vi "Laser 1 Operations L2.vi"(8 "Error in":errorcluster caption="Error in (no error)", 10 "Queues Cluster":T1, 11 "UI elements cluster":T2) -> (0 "Error out":errorcluster)   [LabVIEW 2017]
uses:
  Global Variables/General Globals.vi
  Typedefs/XY Stage config cluster.ctl
  Typedefs/Cam VidRec HW config setup cluster.ctl
  Typedefs/Control Sys HW config cluster.ctl
  <vilib>/userdefined/High Color/nirio_resource_hc.ctl
  Typedefs/FPGA input type AC-DC.ctl
  Typedefs/DAQmx physical channels cluster.ctl
  Typedefs/Encoder config cluster.ctl
  Typedefs/Z Stage config cluster.ctl
  Typedefs/Triggers HW config.ctl
  Typedefs/Laser 1 config cluster.ctl
  Typedefs/PreChirper 1 config cluster.ctl
  Typedefs/Microscope Config.ctl
  Typedefs/Laser Power Control HW config.ctl
  Typedefs/Hardware Configuration settings.ctl
  Serial Comms/Visa resource.ctl
  Typedefs/Plane Mode.ctl
  Typedefs/Laser control knob.ctl
  Typedefs/PMT control knob.ctl
  Typedefs/XY Stage_Move.ctl
  Typedefs/Frame Size.ctl
  Typedefs/UI ctrl refs cluster.ctl
  Typedefs/Imaging Param ref.ctl
  User Interface/Queue/Message Queue/Typedefs/Message Cluster.ctl
  Typedefs/Imaging Protocols enum.ctl
  Typedefs/Acquired points count.ctl
  Typedefs/Logging queue element.ctl
  User Interface/Queue/Message Queue/Typedefs/All Message Queues.ctl
panel:
  in  "Wavelength \n(set) [nm]":u16
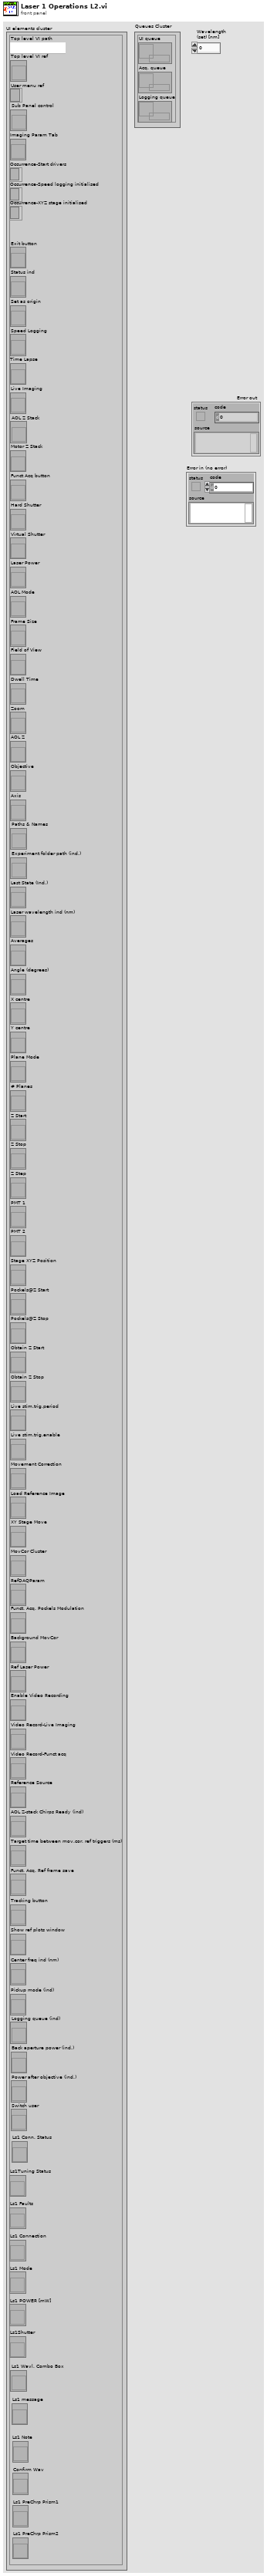
[diagram p1: front panel]
types:
  T1 = typedef "All Message Queues.ctl" = cluster{"UI queue":refnum<queue>, "Acq. queue":refnum<queue>, "Logging queue":refnum<queue>}
  T2 = typedef "UI ctrl refs cluster.ctl" = cluster{"Top level VI path":path, "Top level VI ref":refnum<vi>, "User menu ref":refnum<k9>, "Sub Panel control":refnum<vi>, "Imaging Param Tab":T3, "Occurrence-Start drivers":refnum<k4>, "Occurrence-Speed logging initialised":refnum<k4>, "Occurrence-XYZ stage initialised":refnum<k4>, "Exit button":refnum<vi>, "Status ind":refnum<vi>, "Set as origin":refnum<vi>, "Speed Logging":refnum<vi>, "Time Lapse":refnum<vi>, "Live Imaging":refnum<vi>, "AOL Z Stack":refnum<vi>, "Motor Z Stack":refnum<vi>, "Funct Acq button":refnum<vi>, "Hard Shutter":refnum<vi>, "Virtual Shutter":refnum<vi>, "Laser Power":refnum<vi>, "AOL Mode":refnum<vi>, "Frame Size":refnum<vi>, "Field of View":refnum<vi>, "Dwell Time":refnum<vi>, "Zoom":refnum<vi>, "AOL Z":refnum<vi>, "Objective":refnum<vi>, "Axis":refnum<vi>, "Paths & Names":refnum<vi>, "Experiment folder path (ind.)":refnum<vi>, "Last State (Ind.)":refnum<vi>, "Laser wavelength ind (nm)":refnum<vi>, "Averages":refnum<vi>, "Angle (degrees)":refnum<vi>, "X centre":refnum<vi>, "Y centre":refnum<vi>, "Plane Mode":refnum<vi>, "# Planes":refnum<vi>, "Z Start":refnum<vi>, "Z Stop":refnum<vi>, "Z Step":refnum<vi>, "PMT 1":refnum<vi>, "PMT 2":refnum<vi>, "Stage XYZ Position":refnum<vi>, "Pockels@Z Start":refnum<vi>, "Pockels@Z Stop":refnum<vi>, "Obtain Z Start":refnum<vi>, "Obtain Z Stop":refnum<vi>, "Live stim.trig.period":refnum<vi>, "Live stim.trig.enable":refnum<vi>, "Movement Correction":refnum<vi>, "Load Reference Image":refnum<vi>, "XY Stage Move":refnum<vi>, "MovCor Cluster":refnum<vi>, "RefDAQParam":refnum<vi>, "Funct. Acq. Pockels Modulation":refnum<vi>, "Background MovCor":refnum<vi>, "Ref Laser Power":refnum<vi>, "Enable Video Recording":refnum<vi>, "Video Record-Live Imaging":refnum<vi>, "Video Record-Funct acq":refnum<vi>, "Reference Source":refnum<vi>, "AOL Z-stack Chirps Ready (ind)":refnum<vi>, "Target time between mov.cor. ref triggers (ms)":refnum<vi>, "Funct. Acq. Ref frame save":refnum<vi>, "Tracking button":refnum<vi>, "Show ref plots window":refnum<vi>, "Center freq ind (nm)":refnum<vi>, "Pickup mode (ind)":refnum<vi>, "Logging queue (ind)":refnum<vi>, "Back aperture power (ind.)":refnum<vi>, "Power after objective (ind.)":refnum<vi>, "Switch user":refnum<vi>, "Ls1 Conn. Status":refnum<vi>, "Ls1Tuning Status":refnum<vi>, "Ls1 Faults":refnum<vi>, "Ls1 Connection":refnum<vi>, "Ls1 Mode":refnum<vi>, "Ls1 POWER [mW]":refnum<vi>, "Ls1Shutter":refnum<vi>, "Ls1 Wavl. Combo Box":refnum<vi>, "Ls1 message":refnum<vi>, "Ls1 Note":refnum<vi>, "Confirm Wav":refnum<vi>, "Ls1 PreChrp Prism1":refnum<vi>, "Ls1 PreChrp Prism2":refnum<vi>}
  T3 = typedef "Imaging Param ref.ctl" = refnum<vi>
  T4 = typedef "Hardware Configuration settings.ctl" = cluster{"Computer MAC address":string, "XY Stage":T5, "Cam VidRec":T6, "Control Sys. HW config":T7, "DAQ FPGA HW Config":cluster{"Target":T8, "input card type":T9}, "DAQmx Chan":T10, "Encoder":T11, "Z Stage config cluster":T12, "Trigger HW config":T13, "Externalise Triggers":bool, "MC Supported":bool, "Laser 1 config cluster":T14, "Prechirper 1 config cluster":T15, "Microscope Config":T16, "Laser Power Control HW config":T17, "No of AOD":u8, "Dev. PC":bool}
  T5 = typedef "XY Stage config cluster.ctl" = cluster{"COM port":refnum<visa-resource-name>, "XY stage available":bool, "Baudrate":i32, "Type":string}
  T6 = typedef "Cam VidRec HW config setup cluster.ctl" = cluster{"DO flag-Video record":tag, "DO flag-Trial start":tag, "VidRec available":bool}
  T7 = typedef "Control Sys HW config cluster.ctl" = cluster{"Ctrl system MAC address":string, "Control system.Network adapter name":string, "Ctrl FPGA available":bool}
  T8 = typedef "nirio_resource_hc.ctl" = tag
  T9 = typedef "FPGA input type AC-DC.ctl" = enum16{"AC Card", "DC Card"}
  T10 = typedef "DAQmx physical channels cluster.ctl" = cluster{"Pockels AO":tag, "Hard shutter AO":tag, "PMT AOs":tag, "Power meter AI":tag}
  T11 = typedef "Encoder config cluster.ctl" = cluster{"IP address":string, "Port":u16, "Encoder available":bool, "Wheel radius (cm)":dbl}
  T12 = typedef "Z Stage config cluster.ctl" = cluster{"COM port":refnum<visa-resource-name>, "Z stage available":bool, "Baudrate":i32, "Type":string}
  T13 = typedef "Triggers HW config.ctl" = cluster{"Available Device List":i32, "Device Address":string}
  T14 = typedef "Laser 1 config cluster.ctl" = cluster{"COM port":refnum<visa-resource-name>, "Laser 1 available":bool, "Baud Rate":i32, "Type":string}
  T15 = typedef "PreChirper 1 config cluster.ctl" = cluster{"COM port":refnum<visa-resource-name>, "Prechirper 1 \navailable":bool, "Baud Rate":i32, "Type":string}
  T16 = typedef "Microscope Config.ctl" = cluster{"ID":string, "Type":string}
  T17 = typedef "Laser Power Control HW config.ctl" = cluster{"Laser Power Control":string, "Laser Power Modulation Control":string}
  T18 = enum16{"Initialise Connections", "Initialise system", "Check Status", "Open/Close Shutter", "Set wavelength", "Close"}
  T19 = typedef "Visa resource.ctl" = cluster{"VISA resource name":refnum<visa-resource-name>, "baud rate":u32}
  T20 = enum16{"Initialise", "Disable Controls", "Enable Controls", "Update Connection Info", "Update Laser Warning", "Update Laser status", "Update Laser Wav.", "Update prechiper settings"}
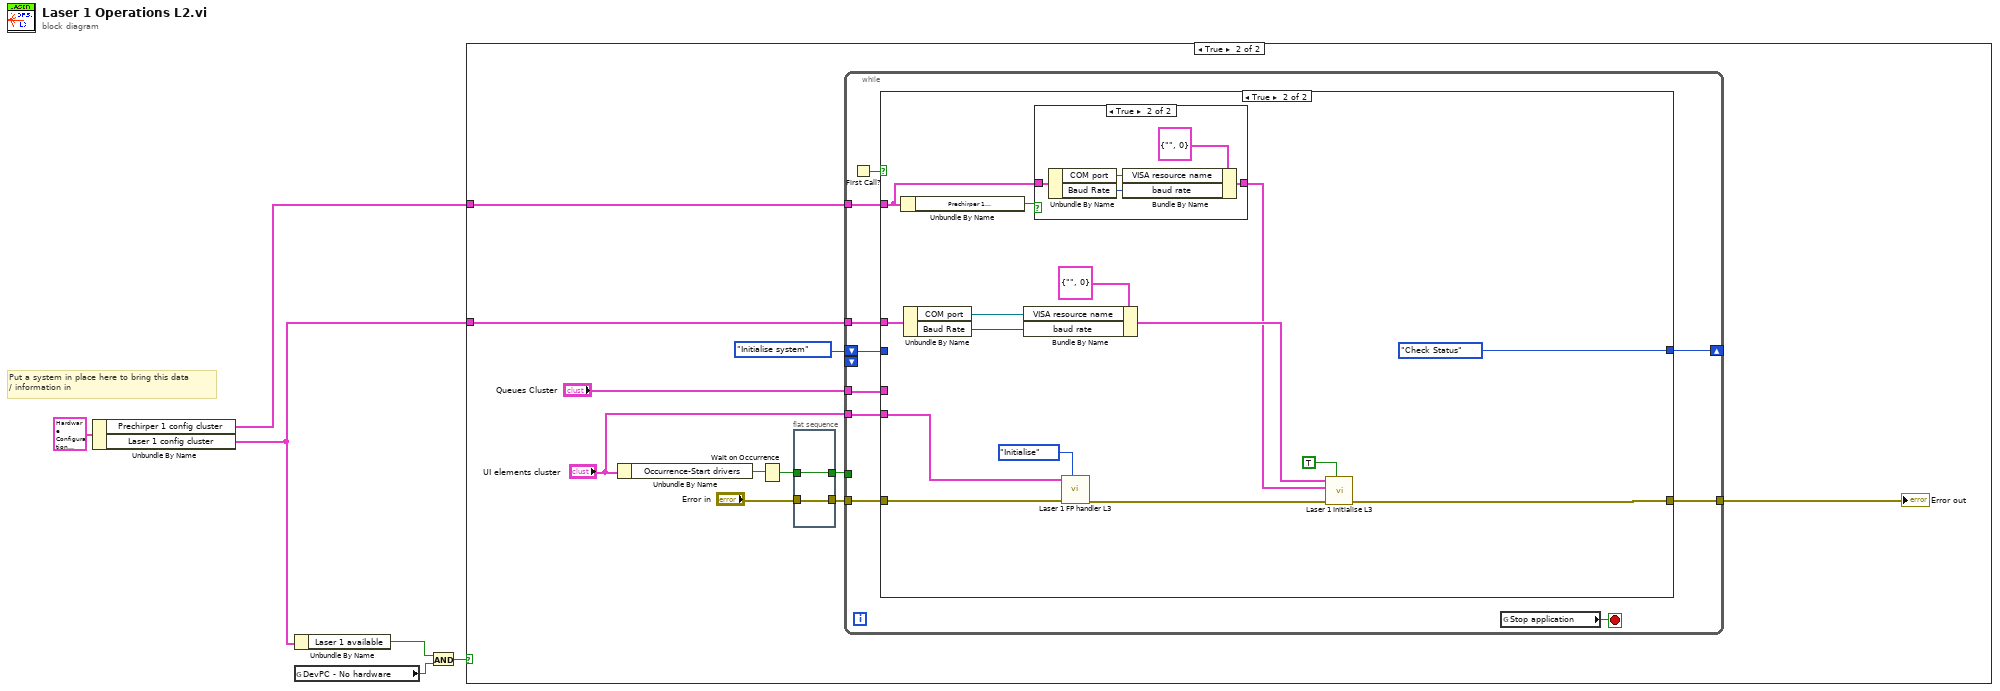
[diagram p0: block diagram]
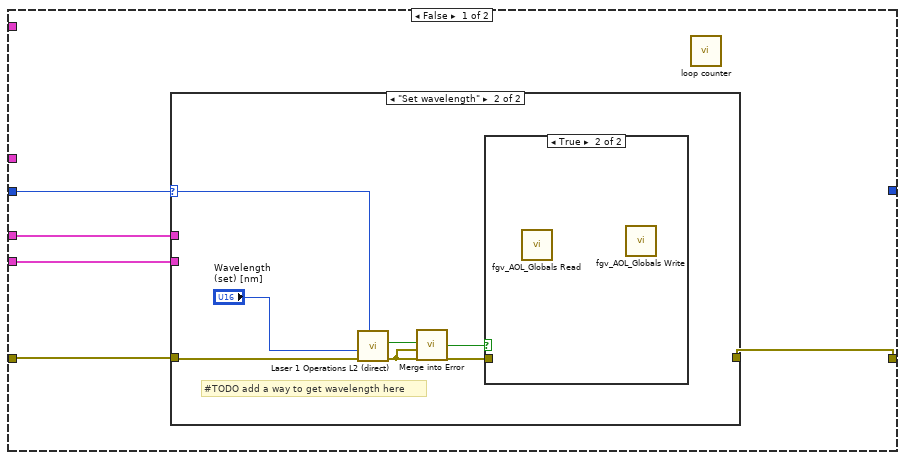
[diagram p3: hidden frame]
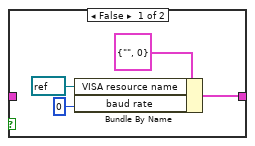
[diagram p6: hidden frame]
diagram:
  # "Put a system in place here to bring this data\n/ information in"
  n1 = Unbundle By Name(T4 {"Computer MAC address"="", "XY Stage"={"COM port"="", "XY stage available"=FALSE, "Baudrate"=0, "Type"=""}, "Cam VidRec"={"DO flag-Video record"="", "DO flag-Trial start"="", "VidRec available"=FALSE}, "Control Sys. HW config"={"Ctrl system MAC address"="", "Control system.Network adapter name"="", "Ctrl FPGA available"=FALSE}, "DAQ FPGA HW Config"={"Target"="RIO0", "input card type"=enum."AC Card"}, "DAQmx Chan"={"Pockels AO"="", "Hard shutter AO"="", "PMT AOs"="", "Power meter AI"=""}, "Encoder"={"IP address"="224.0.1.103", "Port"=7000, "Encoder available"=FALSE, "Wheel radius (cm)"=16.0}, "Z Stage config cluster"={"COM port"="COM7", "Z stage available"=FALSE, "Baudrate"=0, "Type"=""}, "Trigger HW config"={"Available Device List"=0, "Device Address"=""}, "Externalise Triggers"=FALSE, "MC Supported"=FALSE, "Laser 1 config cluster"={"COM port"="COM7", "Laser 1 available"=FALSE, "Baud Rate"=0, "Type"=""}, "Prechirper 1 config cluster"={"COM port"="COM7", "Prechirper 1 \navailable"=FALSE, "Baud Rate"=0, "Type"=""}, "Microscope Config"={"ID"="", "Type"=""}, "Laser Power Control HW config"={"Laser Power Control"="", "Laser Power Modulation Control"=""}, "No of AOD"=0, "Dev. PC"=FALSE} ("Hardware Configuration")) -> ("Prechirper 1 config cluster"=w1:T15, "Laser 1 config cluster"=w5:T14)
  n2 = Unbundle By Name(w5) -> ("Laser 1 available"=w3:bool)
  n3 = global read "General Globals.vi" "DevPC - No hardware"() -> (w4:bool)
  n4 = And(x=w3, y=w4) -> (x .and. y?=w2:bool)
  n5 = case shown="True" w2 {
    tunnel: w5 -> [_ w8]
    tunnel: w1 -> [_ w7]
    frame False {
    }
    frame True {
      n6 = Unbundle By Name("UI elements cluster") -> ("Occurrence-Start drivers"=w17:refnum<k4>)
      n7 = Wait on Occurrence(2:w17) -> (0:w16:bool)  [unwired: 2 in]
      n8 = flat-sequence {
        tunnel: w16 -> [w19]
        tunnel: [w19] -> w13
        tunnel: "Error in" -> [w18]
        tunnel: [w18] -> w14
        frame #0 {
        }
      }
      n9 = while {
        tunnel: w14 -> [w27]
        tunnel: w13 -> [_]
        tunnel: "UI elements cluster" -> [w26]
        tunnel: [w25] -> w11
        shift-right: [w23] -> _
        shift-left: T18."Initialise system" ("Laser Ops actions") -> [w24]
        shift-left: _ -> [_]
        tunnel: "Queues Cluster" -> [w22]
        tunnel: w8 -> [w21]
        tunnel: w7 -> [w20]
        stop <- w29 stop-if-true
        n10 = First Call?() -> (First Call?: T/F=w28:bool)
        n11 = case shown="True" w28 {
          tunnel: w27 -> [w34 w54]
          tunnel: w26 -> [w32 w51]
          tunnel: [w30 w50] -> w25
          tunnel: w24 -> [w33 _]
          tunnel: [_ T18."Check Status" ("Laser Ops actions")] -> w23
          tunnel: w22 -> [w31 _]
          tunnel: w21 -> [_ w48]
          tunnel: w20 -> [_ w42]
          frame False {
            n12 = case shown="\"Set wavelength\"" w33 {
              selector: w33 -> [_ w39]
              tunnel: w34 -> [_ w38]
              tunnel: w32 -> [_ _]
              tunnel: w31 -> [_ _]
              tunnel: [_ _] -> w30
              frame Default {
              }
              frame "Set wavelength" {
                # "#TODO add a way to get wavelength here"
                n13 = call "Laser 1 Operations L2 (direct).vi"("Laser Ops\n actions"=w39, "error in (no error)"=w38, "Wavelength \n(set) [nm]"="Wavelength \n(set) [nm]") -> ("error out"=w37:errorcluster, "Resp Validated"=w40:bool)  [unwired: 4 in, 3 out]
                n14 = call "Merge into Error.vi"("Boolean in"=w40, "error in (no error)"=w37) -> ("Boolean out"=w36:bool)  [unwired: 6 in]
                n15 = case shown="True" w36 {
                  tunnel: w37 -> [_ _]
                  frame False {
                  }
                  frame True {
                    n16 = call "fgv_AOL_Globals Read.vi"() -> ()  [unwired: 9 in, 3 out]
                    n17 = call "fgv_AOL_Globals Write.vi"() -> ()  [unwired: 11 in, 1 out]
                  }
                }
              }
            }
            n18 = call "loop counter.vi"() -> ()  [unwired: 9 in, 1 out]
          }
          frame True {
            n19 = Unbundle By Name(w42) -> ("Prechirper 1 \navailable"=w43:bool)
            n20 = Unbundle By Name(w48) -> ("COM port"=w46:refnum<visa-resource-name>, "Baud Rate"=w45:i32)
            n21 = Bundle By Name(cluster=T19 {"VISA resource name"="", "baud rate"=0} ("Ls1 Visa \nresource"), "VISA resource name"=w46, "baud rate"=w45) -> (w44:T19)
            n22 = case shown="True" w43 {
              tunnel: w42 -> [_ w61]
              tunnel: [w56 w60] -> w41
              frame False {
                n23 = Bundle By Name(cluster=T19 {"VISA resource name"="", "baud rate"=0} ("Ls1 Visa \nresource"), "VISA resource name"=refnum<visa-resource-name> refnum, "baud rate"=u32 0) -> (w56:T19)
              }
              frame True {
                n24 = Unbundle By Name(w61) -> ("COM port"=w63:refnum<visa-resource-name>, "Baud Rate"=w62:i32)
                n25 = Bundle By Name(cluster=T19 {"VISA resource name"="", "baud rate"=0} ("Ls1 Visa \nresource"), "VISA resource name"=w63, "baud rate"=w62) -> (w60:T19)
              }
            }
            n26 = call "Laser 1 FP handler L3.vi"("FP Ops"=T20."Initialise", "Error in"=w54, "UI elements cluster"=w51) -> ("Error out"=w53:errorcluster)  [unwired: 7 in, 1 out]
            n27 = call "Laser 1 Initialise L3.vi"("from FGV ?"=TRUE, "Error in"=w53, "PreChrp1 \nVisa resource"=w41, "Ls1 Visa \nresource"=w44) -> ("Error out"=w50:errorcluster)  [unwired: 7 in]
          }
        }
        n28 = global read "General Globals.vi" "Stop application"() -> (w29:bool)
      }
      "Error out" <- w11
    }
  }
